vi "convert custom error ring to error code (sub-vi).vi"(4 "custom error ring":T1 items=["parse_failure"=-8001, "arduino_failure"=-8002, "manifold_config_value_error"=-8101, "odor_config_value_error"=-8102]) -> (1 "error code":i32)   [LabVIEW 2021]
uses:
  type-defs/project_custom_error_codes_ring (type def).ctl
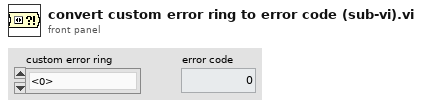
[diagram p1: front panel]
types:
  T1 = typedef "project_custom_error_codes_ring (type def).ctl" = i32
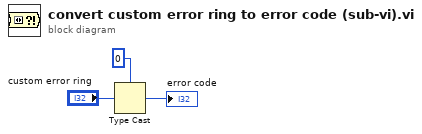
[diagram p0: block diagram]
diagram:
  n1 = Type Cast(type=0 ("code"), x="custom error ring") -> (*(type *) &x=→"error code":i32)
